vi "Create.vi"(8 "error in (no error)":errorcluster, 11 "User Interface in":refnum<class "User Interface.lvclass">) -> (0 "error out":errorcluster, 3 "User Interface out":refnum<class "User Interface.lvclass">)   [LabVIEW 2017, in "DSF Core.lvlib" / "User Interface.lvclass"]
uses:
  User Interface.lvclass
  User Interface.lvclass/User Interface.ctl
  Default User Interface.vi
  User Interface Events/User Interface Events.lvclass
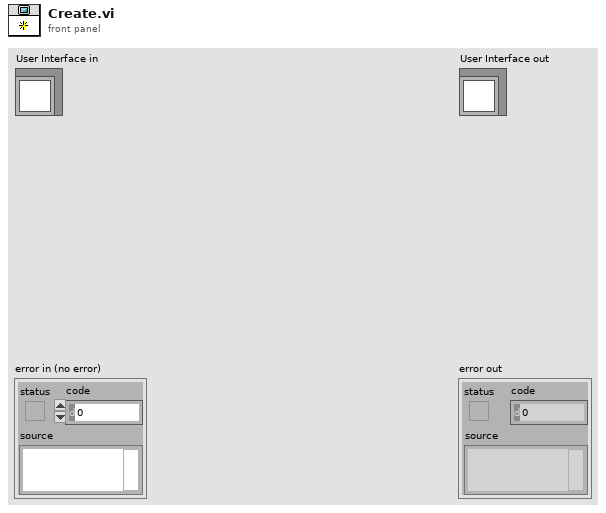
[diagram p1: front panel]
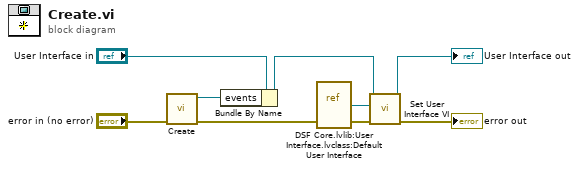
[diagram p0: block diagram]
diagram:
  n1 = call "Create.vi"("error in (no error)"="error in (no error)") -> ("error out"=w5:errorcluster, "User Interface Events out"=w7:refnum<class "User Interface Events.lvclass">)  [unwired: 9 in]
  n2 = Bundle By Name(cluster="User Interface in", "events"=w7) -> (w3:refnum<class "User Interface.lvclass">)
  n3 = vi-ref "DSF Core.lvlib:User Interface.lvclass:Default User Interface.vi"() -> (w1:refnum<vi>)
  n4 = call "Set User Interface VI.vi"("error in (no error)"=w5, "vi"=w1, "User Interface in"=w3) -> ("error out"=→"error out":errorcluster, "User Interface out"=→"User Interface out":refnum<class "User Interface.lvclass">)  [unwired: 7 in]
